vi "6221_write_waveform.vi"(5 "Counter Task In":refnum<k21>, 6 "Error In":errorcluster, 7 "Control Reference Cluster Input":T1, 8 "Waveform Task In":refnum<k21>, 9 "ODT Params":T2={"Waveform Parameters"=[[{"Initial Value"=1.0, "Final Value"=1.0, "Tau"=1.0, "Eta"=10.0, "Nickname"="Channel 0 A", "Function Type"=enum."Power Law", "Conversion"=enum."Volts", "Constant"=0.0}, {"Initial Value"=0.0, "Final Value"=0.0, "Tau"=0.0, "Eta"=0.0, "Nickname"="Channel 0 B", "Function Type"=enum."Power Law", "Conversion"=enum."Volts", "Constant"=0.0}, {"Initial Value"=0.0, "Final Value"=0.0, "Tau"=0.0, "Eta"=0.0, "Nickname"="Channel 0 C", "Function Type"=enum."Power Law", "Conversion"=enum."Volts", "Constant"=0.0}, {"Initial Value"=0.0, "Final Value"=0.0, "Tau"=0.0, "Eta"=0.0, "Nickname"="Channel 0 D", "Function Type"=enum."Power Law", "Conversion"=enum."Volts", "Constant"=0.0}], [{"Initial Value"=0.0, "Final Value"=0.0, "Tau"=0.0, "Eta"=0.0, "Nickname"="Channel 1 A", "Function Type"=enum."Power Law", "Conversion"=enum."Volts", "Constant"=0.0}, {"Initial Value"=0.0, "Final Value"=0.0, "Tau"=0.0, "Eta"=0.0, "Nickname"="Channel 1 B", "Function Type"=enum."Power Law", "Conversion"=enum."Volts", "Constant"=0.0}, {"Initial Value"=0.0, "Final Value"=0.0, "Tau"=0.0, "Eta"=0.0, "Nickname"="Channel 1 C", "Function Type"=enum."Power Law", "Conversion"=enum."Volts", "Constant"=0.0}, {"Initial Value"=0.0, "Final Value"=0.0, "Tau"=0.0, "Eta"=0.0, "Nickname"="Channel 1 D", "Function Type"=enum."Power Law", "Conversion"=enum."Volts", "Constant"=0.0}]], "Active Phases"=[TRUE, FALSE, FALSE, FALSE], "Active Channels"=[TRUE, FALSE], "Phase Times (s)"=[0.001, 0.0, 0.0, 0.0], "Active Device"="6221_ODT", "Trigger Channel"="/6221_ODT/PFI0", "Evaporation Phase"=0.0, "Evaporation Channel"=0.0} {"Evaporation Channel" min=0.0 max=1.0 step=1.0; "Evaporation Phase" min=0.0 max=4.0 step=1.0; "Phase Times (s)" format="%#_6p"}) -> (0 "Error Out":errorcluster, 1 "Counter Task Out":refnum<k21>, 2 "Waveform Task Out":refnum<k21>)   [LabVIEW 2016]
uses:
  6221_panel.ctl
  Controls/6221/6221_waveform_input.ctl
  6221_waveform_param.ctl
  6733_Red_MOT/Neutral_voltage_conversion_control.ctl
  6221_states.ctl
  <vilib>/DAQmx/write.llb/DAQmx Write (Analog 1D DBL NChan 1Samp).vi
  <vilib>/DAQmx/write.llb/DAQmx Write (Analog 1D Wfm NChan NSamp).vi
  <vilib>/DAQmx/create/channels.llb/DAQmx Create Channel (AO-Voltage-Basic).vi
  <vilib>/DAQmx/miscellaneous.llb/DAQmx Fill In Error Info.vi
  <vilib>/Waveform/WDTOps.llb/WDT Append Waveforms DBL.vi
  <vilib>/Waveform/WDTOps.llb/WDT Scale Delta t DBL.vi
  <vilib>/DAQmx/configure/timing.llb/DAQmx Timing (Sample Clock).vi
  <vilib>/DAQmx/create/channels.llb/DAQmx Create Channel (CO-Pulse Generation-Frequency).vi
  <vilib>/DAQmx/configure/timing.llb/DAQmx Timing (Implicit).vi
  <vilib>/DAQmx/configure/trigger.llb/DAQmx Start Trigger (Digital Edge).vi
  <resource>/objmgr/daqmx.rc
panel:
  out "Waveform Graph":waveform(dbl)[](graph)
  out "Samples Written":dbl
  out "Waveforms":waveform(dbl)[](array[waveform])
  out "Sample Rate":dbl
  out "Max Sample Rate":dbl
  out "Total Time":dbl
  out "Inactive Channels":tag[](array[tag])
  out "Active Channels":tag[](array[tag])
  out "# Inactive Channels":i32
  out "# Active Channels":i32
  out "AO.Voltage.Rngs":dbl[](array[numeric])
  out "AO.PhysicalChans":tag[](array[tag])
  out "Active Device":tag
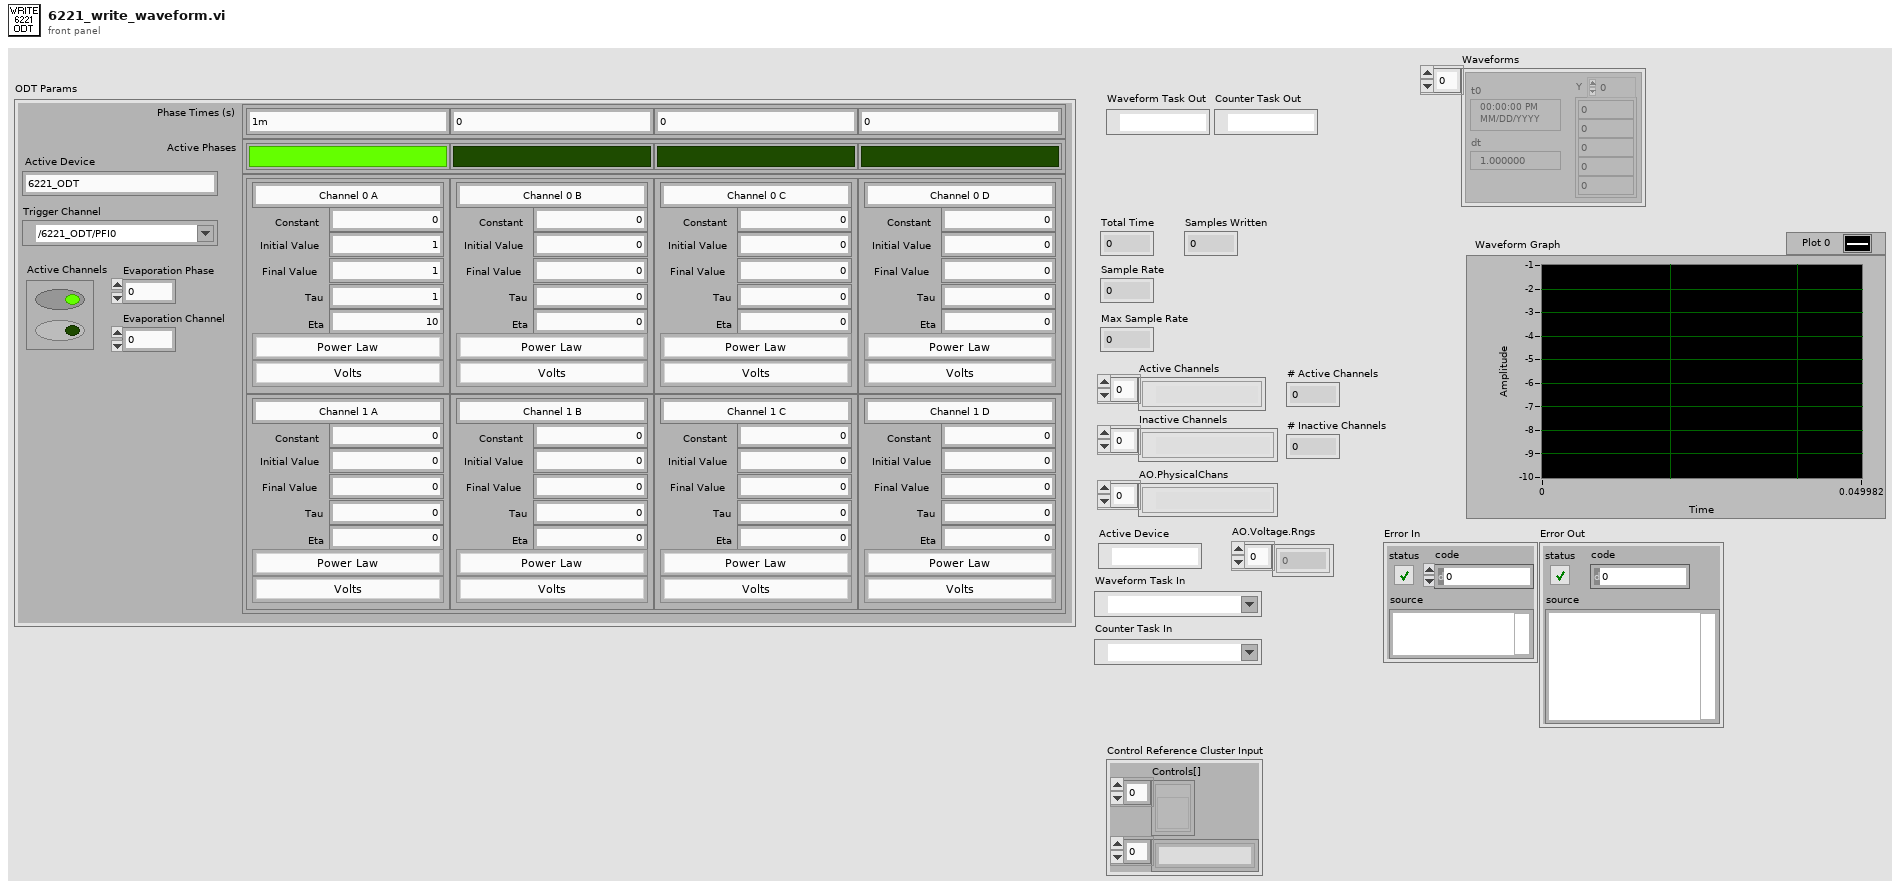
[diagram p1: front panel]
types:
  T1 = cluster{"Controls[]":refnum<vi>[], "Control Names":string[]}
  T2 = typedef "6221_panel.ctl" = cluster{"Waveform Parameters":T3, "Active Phases":bool[], "Active Channels":bool[], "Phase Times (s)":dbl[], "Active Device":string, "Trigger Channel":tag, "Evaporation Phase":dbl, "Evaporation Channel":dbl}
  T3 = typedef "6221_waveform_input.ctl" = T4[][]
  T4 = typedef "6221_waveform_param.ctl" = cluster{"Initial Value":dbl, "Final Value":dbl, "Tau":dbl, "Eta":dbl, "Nickname":string, "Function Type":enum16{"Constant", "Power Law", "Evap - Calc Tau", "Evaporation Formula", "Tanh", "Exponential"}, "Conversion":T5, "Constant":dbl}
  T5 = typedef "Neutral_voltage_conversion_control.ctl" = enum16{"Volts", "B Field Grad (G/cm)", "Red Boson Cntr Freq (MHz)", "Red Boson Dither Amp (kHz)", "Red Boson Power (mW)", "Red 87 Trap Cntr Freq (MHz)", "Red 87 Trap Dither Amp (kHz)", "Red 87 Trap Power (mW)", "Red 87 Stir Cntr Freq (MHz)", "Red 87 Stir Dither Amp (kHz)", "Red 87 Stir Power (mW)", "ODT Sheet Trap Power (W)", "ODT Loading Trap Power (W)"}
  T6 = typedef "6221_states.ctl" = enum16{"Update Front Panel", "Write to Cards", "Check for Problems", "Write Waveforms", "Maximize Samples / Channel", "Clear Old Tasks", "Get Active/Inactive Channels", "Get Device Information", "Initialize"}
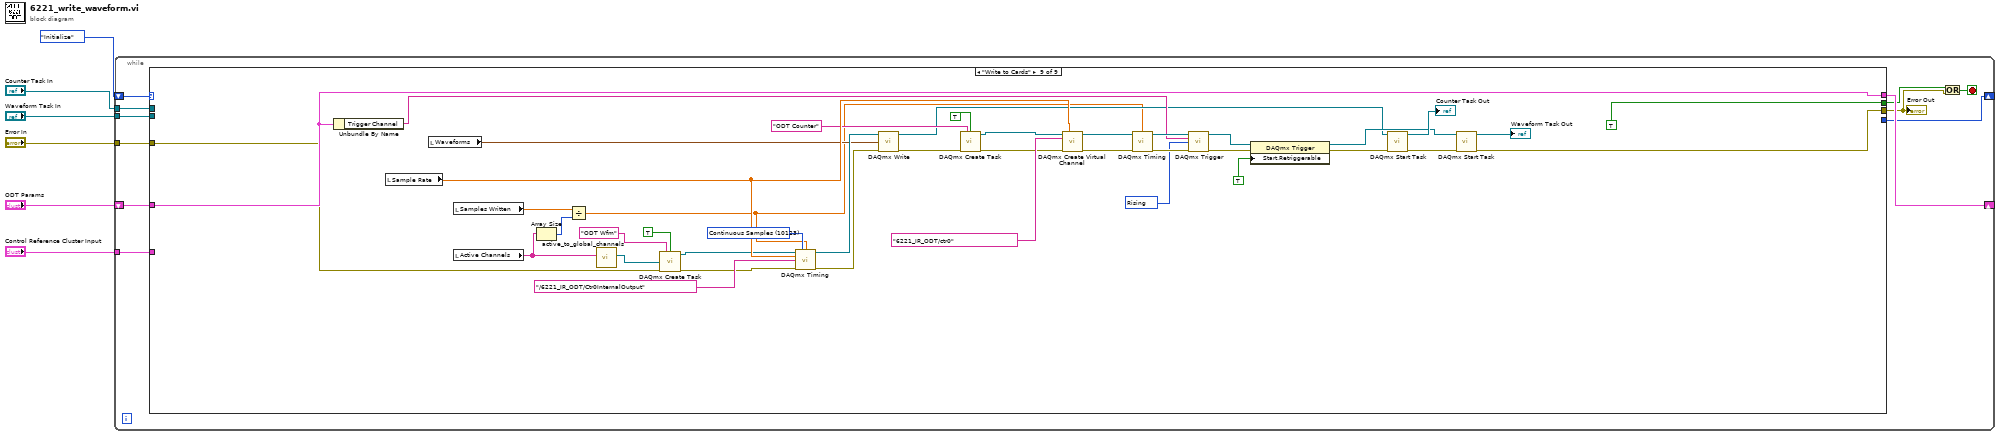
[diagram p0: block diagram]
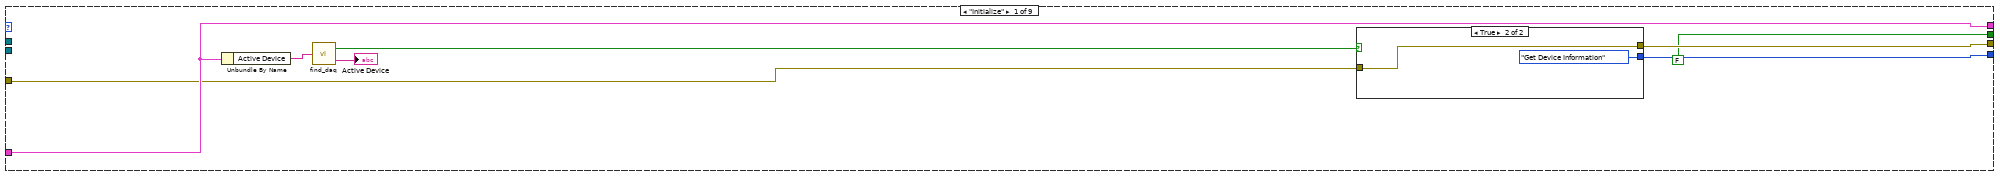
[diagram p2: hidden frame]
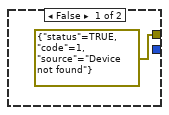
[diagram p3: hidden frame]
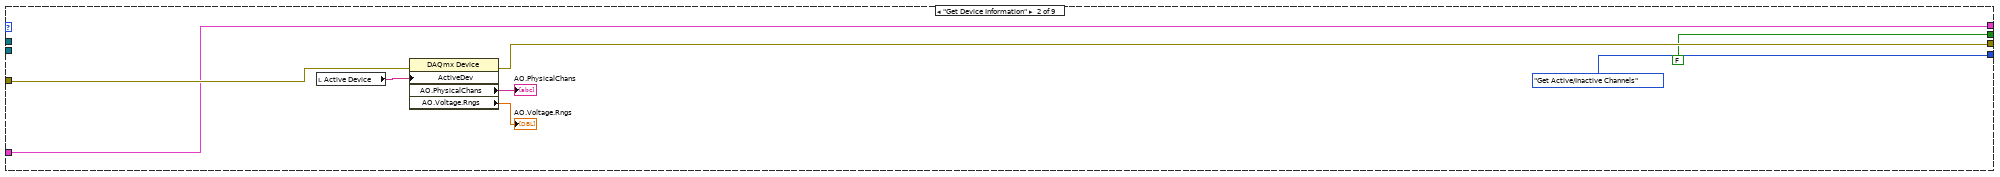
[diagram p4: hidden frame]
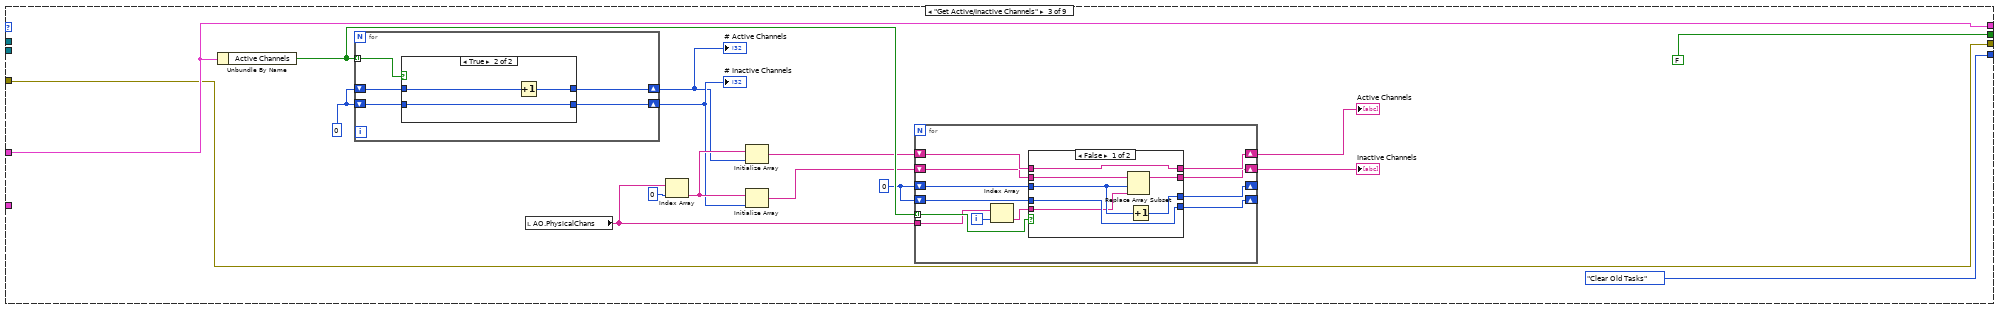
[diagram p5: hidden frame]
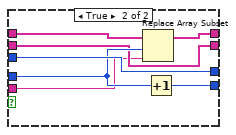
[diagram p6: hidden frame]
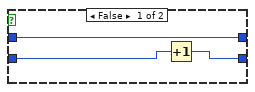
[diagram p7: hidden frame]
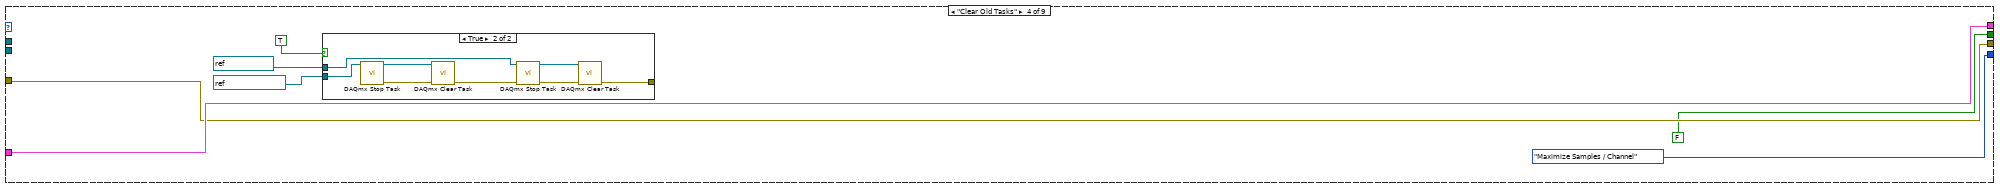
[diagram p8: hidden frame]
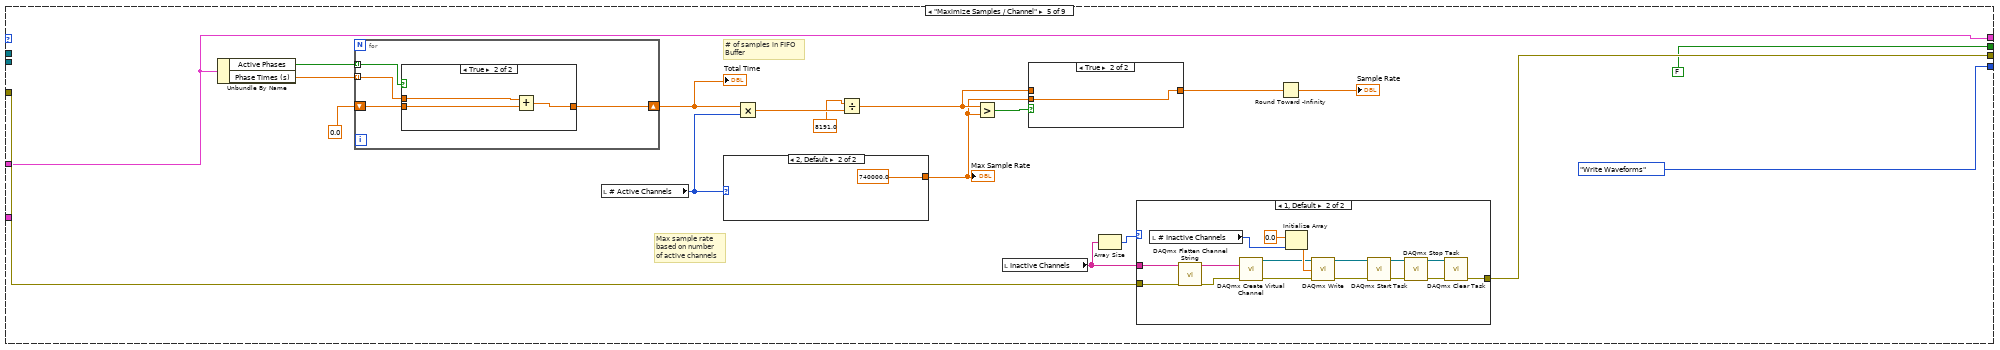
[diagram p10: hidden frame]
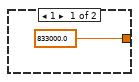
[diagram p13: hidden frame]
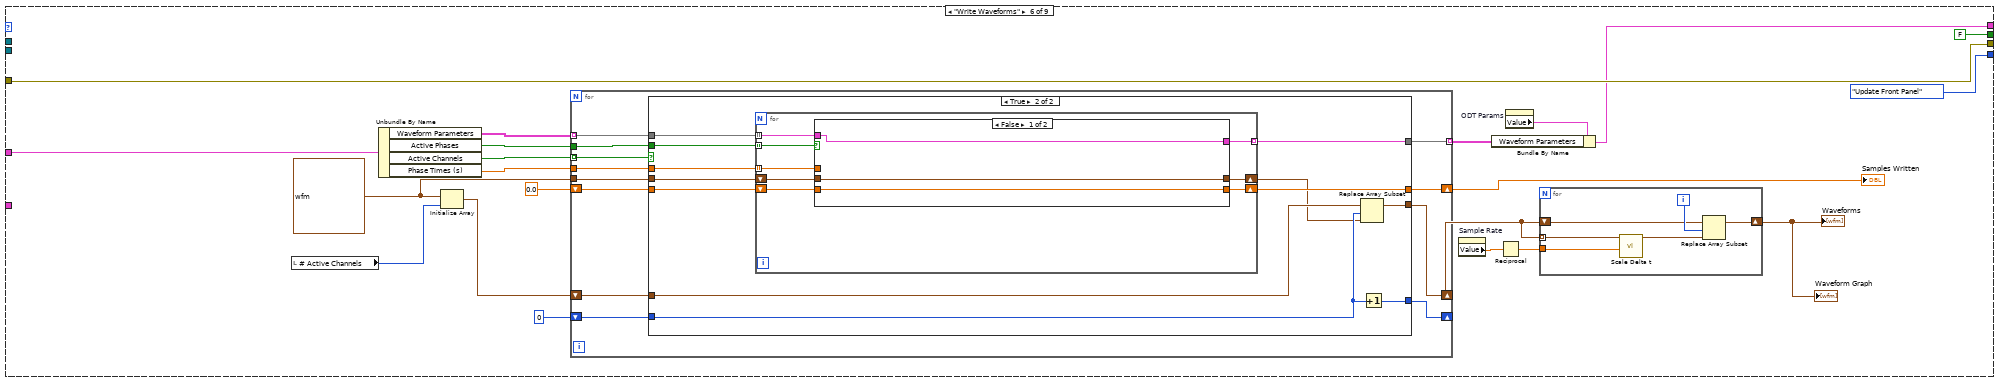
[diagram p15: hidden frame]
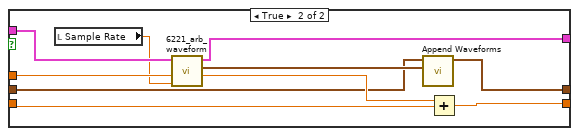
[diagram p17: hidden frame]
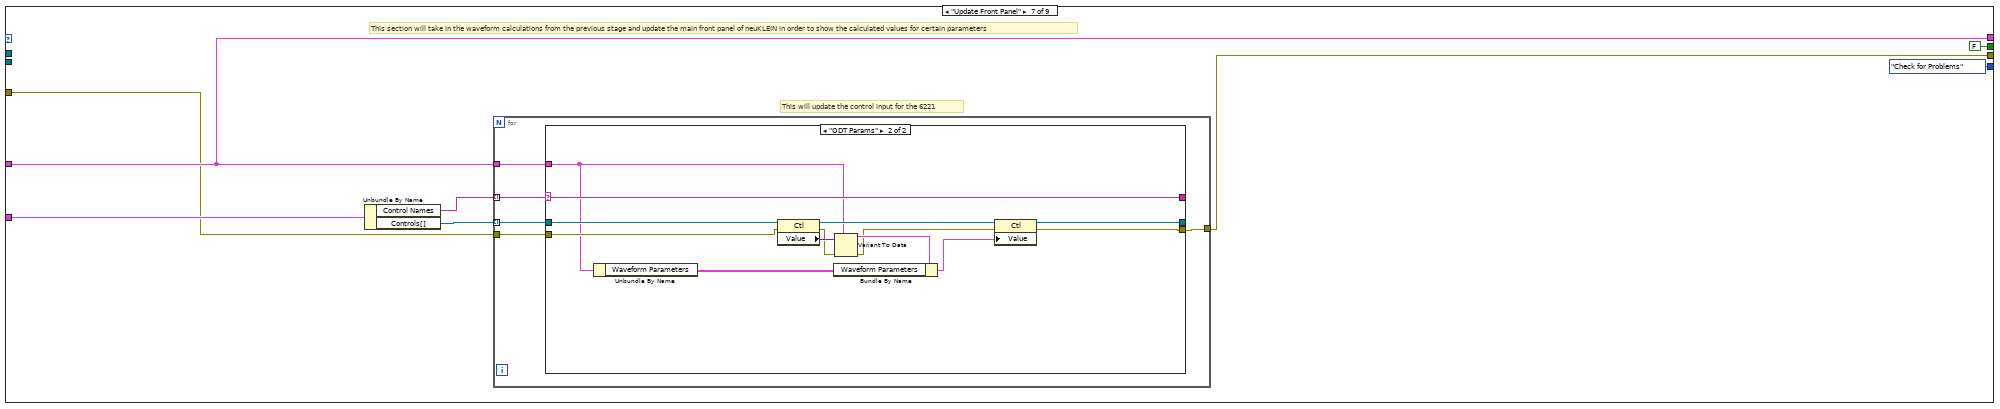
[diagram p18: hidden frame]
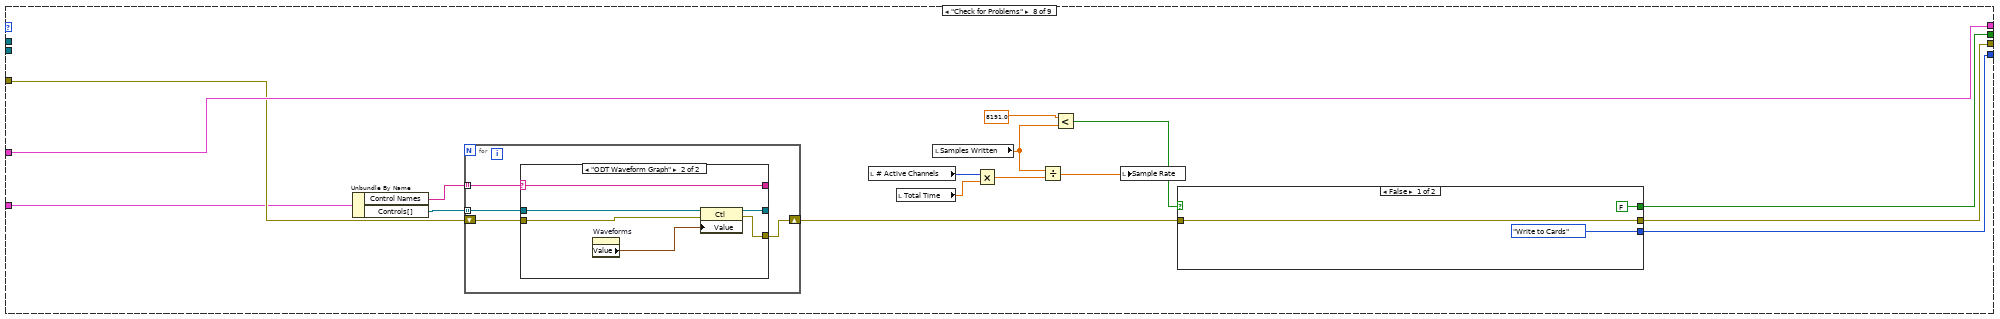
[diagram p20: hidden frame]
diagram:
  n1 = while {
    shift-right: [w14] -> _
    shift-left: 6221_states."Initialize" -> [w17]
    shift-right: [w15] -> _
    shift-left: "ODT Params" -> [w16]
    tunnel: "Error In" -> [w13]
    tunnel: "Waveform Task In" -> [w9]
    tunnel: "Counter Task In" -> [w8]
    tunnel: "Control Reference Cluster Input" -> [w7]
    stop <- w11 stop-if-true
    n2 = case shown="\"Write to Cards\"" w17 {
      tunnel: w16 -> [w25 w32 w52 w96 w120 w160 w232 w273 w313]
      tunnel: [w25 w32 w52 w96 w120 w153 w232 w273 w313] -> w15
      tunnel: [w21 6221_states."Get Active/Inactive Channels" 6221_states."Clear Old Tasks" 6221_states."Maximize Samples / Channel" 6221_states."Write Waveforms" 6221_states."Update Front Panel" 6221_states."Check for Problems" w265 _] -> w14
      tunnel: w13 -> [w20 w35 w50 w94 w123 w173 w231 w259 w310]
      tunnel: [w19 w31 w50 w94 w122 w173 w230 w263 w315] -> w10
      tunnel: [FALSE FALSE FALSE FALSE FALSE FALSE FALSE w264 TRUE] -> w12
      tunnel: w9 -> [_ _ _ _ _ _ _ _ _]
      tunnel: w8 -> [_ _ _ _ _ _ _ _ _]
      tunnel: w7 -> [_ _ _ _ _ _ w233 w258 _]
      frame "Initialize" {
        n3 = Unbundle By Name(w25) -> ("Active Device"=w24:string)
        n4 = call "find_daq.vi"("Device Name"=w24) -> ("Device Present"=w22:bool, "DAQmx Device Name"=→"Active Device":tag)
        n5 = case shown="True" w22 {
          tunnel: [_ 6221_states."Get Device Information"] -> w21
          tunnel: w20 -> [_ w27]
          tunnel: [errorcluster {"status"=TRUE, "code"=1, "source"="Device not found"} ("Error In") w27] -> w19
          frame False {
          }
          frame True {
          }
        }
      }
      frame "Get Device Information" {
        n6 = local read "Active Device"() -> (w36:tag)
        n7 = property class="DAQmx Device"(error in=w35, "ActiveDev"=w36) -> (error out=w31:errorcluster, "AO.PhysicalChans"=→"AO.PhysicalChans":tag[], "AO.Voltage.Rngs"=→"AO.Voltage.Rngs":dbl[])  [unwired: 1 in, 1 out]
      }
      frame "Get Active/Inactive Channels" {
        w43 = 0
        w37 = 0
        n8 = Unbundle By Name(w52) -> ("Active Channels"=w49:bool[])
        n9 = for {
          tunnel: w49 -> [w83] mode=indexing
          shift-right: [w79] -> w45
          shift-left: w37 -> [w82]
          shift-right: [w80] -> w44
          shift-left: w37 -> [w81]
          n10 = case shown="True" w83 {
            tunnel: w82 -> [w84 w87]
            tunnel: w81 -> [w86 w89]
            tunnel: [w86 w88] -> w80
            tunnel: [w85 w87] -> w79
            frame False {
              n11 = Increment(x=w84) -> (x+1=w85:i32)
            }
            frame True {
              n12 = Increment(x=w89) -> (x+1=w88:i32)
            }
          }
        }
        "# Active Channels" <- w44
        "# Inactive Channels" <- w45
        n13 = local read "AO.PhysicalChans"() -> (w48:tag[])
        n14 = Index Array(array=w48, index=0) -> (element=w46:tag)
        n15 = Initialize Array(w46, w44) -> (w41:tag[])
        n16 = Initialize Array(w46, w45) -> (w42:tag[])
        n17 = for {
          tunnel: w49 -> [w64] mode=indexing
          tunnel: w48 -> [w62]
          shift-right: [w53] -> w39
          shift-left: w42 -> [w54]
          shift-right: [w56] -> w40
          shift-left: w41 -> [w57]
          shift-right: [w58] -> _
          shift-left: w43 -> [w60]
          shift-right: [w55] -> _
          shift-left: w43 -> [w59]
          i -> [w63]
          n18 = Index Array(array=w62, index=w63) -> (element=w61:tag)
          n19 = case shown="False" w64 {
            tunnel: w61 -> [w65 w72]
            tunnel: w60 -> [w71 w75]
            tunnel: w59 -> [w68 w76]
            tunnel: [w71 w74] -> w58
            tunnel: w57 -> [w69 w78]
            tunnel: [w69 w77] -> w56
            tunnel: [w70 w76] -> w55
            tunnel: w54 -> [w67 w73]
            tunnel: [w66 w73] -> w53
            frame False {
              n20 = Replace Array Subset(array=w67, new element=w65, index=w68) -> (w66:tag[])
              n21 = Increment(x=w68) -> (x+1=w70:i32)
            }
            frame True {
              n22 = Replace Array Subset(array=w78, new element=w72, index=w75) -> (w77:tag[])
              n23 = Increment(x=w75) -> (x+1=w74:i32)
            }
          }
        }
        "Active Channels" <- w40
        "Inactive Channels" <- w39
      }
      frame "Clear Old Tasks" {
        n24 = case shown="True" TRUE {
          tunnel: [_ w99] -> _
          tunnel: refnum<k21> "ODT Counter" ("Waveform Task In") -> [_ w98]
          tunnel: refnum<k21> "ODT Wfm" ("Counter Task In") -> [_ w97]
          frame False {
          }
          frame True {
            n25 = call <vilib>:"DAQmx Stop Task.vi"("task/channels in"=w98) -> ("task out"=w103:refnum<k21>, "error out"=w104:errorcluster)  [unwired: 13 in]
            n26 = call <vilib>:"DAQmx Clear Task.vi"("task in"=w103, "error in"=w104) -> ("error out"=w100:errorcluster)  [unwired: 13 in]
            n27 = call <vilib>:"DAQmx Stop Task.vi"("task/channels in"=w97, "error in"=w100) -> ("task out"=w102:refnum<k21>, "error out"=w101:errorcluster)  [unwired: 12 in]
            n28 = call <vilib>:"DAQmx Clear Task.vi"("task in"=w102, "error in"=w101) -> ("error out"=w99:errorcluster)  [unwired: 13 in]
          }
        }
      }
      frame "Maximize Samples / Channel" {
        # "Max sample rate\nbased on number\nof active channels"
        # "# of samples in FIFO\nBuffer"
        n29 = Unbundle By Name(w120) -> ("Active Phases"=w118:bool[], "Phase Times (s)"=w119:dbl[])
        n30 = for {
          tunnel: w119 -> [w147] mode=indexing
          tunnel: w118 -> [w148] mode=indexing
          shift-right: [w145] -> w116
          shift-left: 0.0 -> [w146]
          n31 = case shown="True" w148 {
            tunnel: w147 -> [_ w150]
            tunnel: w146 -> [w149 w152]
            tunnel: [w149 w151] -> w145
            frame False {
            }
            frame True {
              n32 = Add(x=w150, y=w152) -> (x+y=w151:dbl)
            }
          }
        }
        "Total Time" <- w116
        n33 = local read "# Active Channels"() -> (w113:i32)
        n34 = case shown="2, Default" w113 {
          tunnel: [833000.0 740000.0] -> w110
          frame 1 {
          }
          frame 2, Default {
          }
        }
        "Max Sample Rate" <- w110
        n35 = Multiply(x=w116, y=w113) -> (x*y=w115:dbl)
        n36 = Divide(x=8191.0, y=w115) -> (x/y=w111:dbl)
        n37 = Greater?(x=w111, y=w110) -> (0:w112:bool)
        n38 = local read "Inactive Channels"() -> (w106:tag[])
        n39 = case shown="True" w112 {
          tunnel: w111 -> [w141 _]
          tunnel: w110 -> [_ w142]
          tunnel: [w141 w142] -> w109
          frame False {
          }
          frame True {
          }
        }
        n40 = Array Size(array=w106) -> (size(s)=w105:i32)
        n41 = case shown="1, Default" w105 {
          tunnel: w106 -> [_ w140]
          tunnel: w123 -> [w124 w139]
          tunnel: [w124 w125] -> w122
          frame 0 {
          }
          frame 1, Default {
            n42 = local read "# Inactive Channels"() -> (w134:i32)
            n43 = call <vilib>:"DAQmx Flatten Channel String.vi"("names in"=w140, "error in"=w139) -> ("names out"=w137:string, "error out"=w138:errorcluster)  [unwired: 12 in]
            n44 = call-poly <vilib>:"DAQmx Create Virtual Channel.vi"("physical channels"=w137, "error in"=w138) -> ("task out"=w132:refnum<k21>, "error out"=w136:errorcluster)  [unwired: 12 in]
            n45 = Initialize Array(0.0 ("element"), w134) -> (w133:dbl[])
            n46 = call-poly <vilib>:"DAQmx Write.vi"("task/channels in"=w132, "data"=w133, "error in"=w136) -> ("task out"=w131:refnum<k21>, "error out"=w130:errorcluster)  [unwired: 10 in, 1 out]
            n47 = call <vilib>:"DAQmx Start Task.vi"("task/channels in"=w131, "error in"=w130) -> ("task out"=w129:refnum<k21>, "error out"=w128:errorcluster)  [unwired: 12 in]
            n48 = call <vilib>:"DAQmx Stop Task.vi"("task/channels in"=w129, "error in"=w128) -> ("task out"=w127:refnum<k21>, "error out"=w126:errorcluster)  [unwired: 12 in]
            n49 = call <vilib>:"DAQmx Clear Task.vi"("task in"=w127, "error in"=w126) -> ("error out"=w125:errorcluster)  [unwired: 13 in]
          }
        }
        n50 = Round Toward -Infinity(1:w109) -> (0:→"Sample Rate":dbl)
      }
      frame "Write Waveforms" {
        w162 = waveform(dbl) {"t0"=timestamp(0 s since 1904-01-01), "dt"=1.0, "Y"=[]} ("waveform")
        n51 = local read "# Active Channels"() -> (w171:i32)
        n52 = Unbundle By Name(w160) -> ("Waveform Parameters"=w165:T3, "Active Phases"=w167:bool[], "Active Channels"=w168:bool[], "Phase Times (s)"=w166:dbl[])
        n53 = Initialize Array(w162, w171) -> (w170:waveform(dbl)[])
        n54 = for {
          shift-right: [w189] -> w159
          shift-left: w170 -> [w188]
          shift-right: [w190] -> _
          shift-left: 0 -> [w187]
          tunnel: w168 -> [w191] mode=indexing
          tunnel: w167 -> [w186]
          tunnel: w166 -> [w185]
          tunnel: w165 -> [w184] mode=indexing
          shift-right: [w182] -> w161
          shift-left: 0.0 ("y") -> [w183]
          tunnel: w162 -> [w181]
          tunnel: [w180] -> w154 mode=indexing
          n55 = case shown="True" w191 {
            tunnel: [w194 w207] -> w190
            tunnel: [w193 w206] -> w189
            tunnel: w188 -> [w193 w205]
            tunnel: w187 -> [w194 w204]
            tunnel: w186 -> [_ w203]
            tunnel: w185 -> [_ w202]
            tunnel: w184 -> [w192 w201]
            tunnel: w183 -> [w195 w200]
            tunnel: [w195 w199] -> w182
            tunnel: w181 -> [_ w198]
            tunnel: [w192 w196] -> w180
            frame False {
            }
            frame True {
              n56 = for {
                tunnel: w203 -> [w215] mode=indexing
                tunnel: w202 -> [w213] mode=indexing
                tunnel: w201 -> [w214] mode=indexing
                shift-right: [w211] -> w199
                shift-left: w200 -> [w212]
                shift-right: [w209] -> w197
                shift-left: w198 -> [w210]
                tunnel: [w208] -> w196 mode=indexing
                n57 = case shown="False" w215 {
                  tunnel: w214 -> [w216 w228]
                  tunnel: w213 -> [_ w227]
                  tunnel: w212 -> [w217 w224]
                  tunnel: [w217 w223] -> w211
                  tunnel: w210 -> [w218 w221]
                  tunnel: [w218 w220] -> w209
                  tunnel: [w216 w219] -> w208
                  frame False {
                  }
                  frame True {
                    n58 = local read "Sample Rate"() -> (w226:dbl)
                    n59 = call "6221_arb_waveform.vi"("Waveform Input"=w228, "Phase Time"=w227, "Sample Rate"=w226) -> ("Waveform Output"=w219:T4, "output waveform"=w222:waveform(dbl), "# Samples"=w225:dbl)  [unwired: 5 in]
                    n60 = call-poly <vilib>:"Append Waveforms.vi"("waveform B"=w222, "waveform A"=w221) -> ("waveform out"=w220:waveform(dbl))  [unwired: 8 in, 1 out]
                    n61 = Add(x=w225, y=w224) -> (x+y=w223:dbl)
                  }
                }
              }
              n62 = Replace Array Subset(array=w205, new element=w197, index=w204) -> (w206:waveform(dbl)[])
              n63 = Increment(x=w204) -> (x+1=w207:i32)
            }
          }
        }
        "Samples Written" <- w161
        n64 = property on="Sample Rate" class="DigNum (strict)"() -> ("Value"=w157:dbl)  [unwired: 2 in, 2 out]
        n65 = Reciprocal(x=w157) -> (1/x=w156:dbl)
        n66 = property on="ODT Params" class="Clust (strict)"() -> ("Value"=w155:T2)  [unwired: 2 in, 2 out]
        n67 = Bundle By Name(cluster=w155, "Waveform Parameters"=w154) -> (w153:T2)
        n68 = for {
          tunnel: w159 -> [w179] mode=indexing
          shift-right: [w175] -> w158
          shift-left: w159 -> [w176]
          tunnel: w156 -> [w174]
          i -> [w178]
          n69 = call-poly <vilib>:"Scale Delta t.vi"("scale factor"=w174, "waveform in"=w179) -> ("waveform out"=w177:waveform(dbl))  [unwired: 8 in, 1 out]
          n70 = Replace Array Subset(array=w176, new element=w177, index=w178) -> (w175:waveform(dbl)[])
        }
        "Waveforms" <- w158
        "Waveform Graph" <- w158
      }
      frame "Update Front Panel" {
        # "This will update the control input for the 6221"
        # "This section will take in the waveform calculations from the previous stage and update the main front panel of neuKLEIN in order to show the calculated values for certain parameters"
        n71 = Unbundle By Name(w233) -> ("Control Names"=w235:string[], "Controls[]"=w234:refnum<vi>[])
        n72 = for {
          tunnel: w235 -> [w241] mode=indexing
          tunnel: w234 -> [w240] mode=indexing
          tunnel: w232 -> [w239]
          tunnel: w231 -> [w238]
          tunnel: [w237] -> w230
          n73 = case shown="\"ODT Params\"" w241 {
            selector: w241 -> [w244 w257]
            tunnel: w240 -> [w243 w256]
            tunnel: [w244 w257] -> _
            tunnel: [w243 w252] -> _
            tunnel: w239 -> [_ w245]
            tunnel: w238 -> [w242 w250]
            tunnel: [w242 w247] -> w237
            frame "False", Default {
            }
            frame "ODT Params" {
              n74 = Unbundle By Name(w245) -> ("Waveform Parameters"=w246:T3)
              n75 = property class="Ctl"(reference=w256, error in=w250) -> (reference out=w253:refnum<vi>, error out=w249:errorcluster, "Value"=w255:variant)
              n76 = Variant To Data(error in=w249, type=w245, Variant=w255) -> (data=w254:T2, error out=w248:errorcluster)
              n77 = Bundle By Name(cluster=w254, "Waveform Parameters"=w246) -> (w251:T2)
              n78 = property class="Ctl"(reference=w253, error in=w248, "Value"=w251) -> (reference out=w252:refnum<vi>, error out=w247:errorcluster)
            }
          }
        }
      }
      frame "Check for Problems" {
        n79 = Unbundle By Name(w258) -> ("Control Names"=w261:string[], "Controls[]"=w262:refnum<vi>[])
        n80 = for {
          tunnel: w261 -> [w277] mode=indexing
          shift-right: [w274] -> w260
          shift-left: w259 -> [w275]
          tunnel: w262 -> [w276] mode=indexing
          n81 = case shown="\"ODT Waveform Graph\"" w277 {
            selector: w277 -> [w280 w286]
            tunnel: w276 -> [w279 w283]
            tunnel: [w280 w286] -> _
            tunnel: [w279 w282] -> _
            tunnel: w275 -> [w278 w285]
            tunnel: [w278 w284] -> w274
            frame "False", Default {
            }
            frame "ODT Waveform Graph" {
              n82 = property on="Waveforms" class="Arr (strict)"() -> ("Value"=w281:waveform(dbl)[])  [unwired: 2 in, 2 out]
              n83 = property class="Ctl"(reference=w283, error in=w285, "Value"=w281) -> (reference out=w282:refnum<vi>, error out=w284:errorcluster)
            }
          }
        }
        n84 = local read "# Active Channels"() -> (w270:i32)
        n85 = local read "Total Time"() -> (w271:dbl)
        n86 = local read "Samples Written"() -> (w268:dbl)
        n87 = Multiply(x=w270, y=w271) -> (x*y=w269:dbl)
        n88 = Divide(x=w268, y=w269) -> (x/y=w267:dbl)
        n89 = Less?(x=8191.0, y=w268) -> (x < y?=w266:bool)
        n90 = local write "Sample Rate"(w267) -> ()
        n91 = case shown="False" w266 {
          tunnel: [6221_states."Write to Cards" _] -> w265
          tunnel: [FALSE TRUE] -> w264
          tunnel: [w287 errorcluster {"status"=TRUE, "code"=2, "source"="number of samples to write larger\nthan FIFO buffer capacity"} ("error in (no error)")] -> w263
          tunnel: w260 -> [w287 _]
          frame False {
          }
          frame True {
          }
        }
      }
      frame "Write to Cards" {
        w296 = 10280 items=["Rising"=10280, "Falling"=10171] ("edge")
        w298 = 10123 items=["Finite Samples"=10178, "Continuous Samples"=10123, "Hardware Timed Single Point"=12522] ("sample mode")
        n92 = Unbundle By Name(w313) -> ("Trigger Channel"=w312:tag)
        n93 = local read "Sample Rate"() -> (w314:dbl)
        n94 = local read "Waveforms"() -> (w297:waveform(dbl)[])
        n95 = local read "Samples Written"() -> (w293:dbl)
        n96 = local read "Active Channels"() -> (w295:tag[])
        n97 = Array Size(array=w295) -> (size(s)=w294:i32)
        n98 = Divide(x=w293, y=w294) -> (x/y=w292:dbl)
        n99 = call "active_to_global_channels.vi"("Active Channels"=w295) -> ("Global Channels"=w311:refnum<k21>)  [unwired: 10 in]
        n100 = call <vilib>:"DAQmx Create Task.vi"("new task name"="ODT Wfm", "auto cleanup"=TRUE, "global virtual channels"=w311, "error in"=w310) -> ("task out"=w308:refnum<k21>, "error out"=w309:errorcluster)  [unwired: 10 in]
        n101 = call-poly <vilib>:"DAQmx Timing.vi"("task/channels in"=w308, "sample mode"=w298, "samples per channel"=w292, "rate"=w314, "source"=tag "/6221_IR_ODT/Ctr0InternalOutput", "error in"=w309) -> ("task out"=w328:refnum<k21>, "error out"=w329:errorcluster)  [unwired: 8 in]
        n102 = call-poly <vilib>:"DAQmx Write.vi"("task/channels in"=w328, "data"=w297, "error in"=w329) -> ("task out"=w299:refnum<k21>, "error out"=w306:errorcluster)  [unwired: 10 in, 1 out]
        n103 = call <vilib>:"DAQmx Create Task.vi"("new task name"="ODT Counter", "auto cleanup"=TRUE, "error in"=w306) -> ("task out"=w303:refnum<k21>, "error out"=w304:errorcluster)  [unwired: 11 in]
        n104 = call-poly <vilib>:"DAQmx Create Virtual Channel.vi"("task in"=w303, "frequency"=w314, "counter"=tag "6221_IR_ODT/ctr0", "error in"=w304) -> ("task out"=w325:refnum<k21>, "error out"=w326:errorcluster)  [unwired: 10 in]
        n105 = call-poly <vilib>:"DAQmx Timing.vi"("task/channels in"=w325, "samples per channel"=w292, "error in"=w326) -> ("task out"=w323:refnum<k21>, "error out"=w324:errorcluster)  [unwired: 11 in]
        n106 = call-poly <vilib>:"DAQmx Trigger.vi"("task/channels in"=w323, "source"=w312, "edge"=w296, "error in"=w324) -> ("task out"=w320:refnum<k21>, "error out"=w322:errorcluster)  [unwired: 10 in]
        n107 = property class="DAQmx Trigger"(reference=w320, error in=w322, "Start.Retriggerable"=TRUE) -> (reference out=w300:refnum<k21>, error out=w319:errorcluster)
        n108 = call <vilib>:"DAQmx Start Task.vi"("task/channels in"=w299, "error in"=w319) -> ("task out"=→"Counter Task Out":refnum<k21>, "error out"=w318:errorcluster)  [unwired: 12 in]
        n109 = call <vilib>:"DAQmx Start Task.vi"("task/channels in"=w300, "error in"=w318) -> ("task out"=→"Waveform Task Out":refnum<k21>, "error out"=w315:errorcluster)  [unwired: 12 in]
      }
    }
    "Error Out" <- w10
    n110 = Or(x=w12, y=w10) -> (x .or. y?=w11:bool)
  }
